vi "Actor Core.vi"(8 "error in":errorcluster, 11 "Nested in":refnum<class "Button_transfer.lvclass">) -> (0 "error out":errorcluster, 3 "Actor out":refnum<class "Actor.lvclass">)   [LabVIEW 2025, in "Button_transfer.lvlib" / "Button_transfer.lvclass"]
doc: "(<B>Filename</B>: Actor Framework.lvlib:Actor.lvclass:Actor Core.vi)\n\nReceives messages to the actor, reacts to them, and initiates any error handling that may shut the actor down.\n\nDescendant classes may override this VI to append parallel tasks for the actor to complete while it handles messages. Overrides use the Call Parent Method node."
uses:
  Button_transfer.lvclass
  C:/Program Files (x86)/National Instruments/LabVIEW 2025/vi.lib/ActorFramework/Actor/Actor.lvclass
  <vilib>/ActorFramework/Actor/Actor.lvclass
  A_Actor/A_Actor.lvclass
  Button_transfer Messages/Update_msg_B Msg/Update_msg_B Msg.lvclass
  C:/Users/halstead_rideriver/Documents/Labview_Practice/Tasks_Actor/A_Actor Messages/A_msg Msg/A_msg Msg.lvclass
  B_Actor/B_Actor.lvclass
  Button_transfer Messages/Update_msg_B2 Msg/Update_msg_B2 Msg.lvclass
  C:/Users/halstead_rideriver/Documents/Labview_Practice/Tasks_Actor/B_Actor Messages/B_msg Msg/B_msg Msg.lvclass
  B_Actor/B_Actor.lvclass/B_Actor.ctl
  A_Actor/A_Actor.lvclass/A_Actor.ctl
  <vilib>/ActorFramework/Actor/Actor.lvclass/Actor.ctl
  <vilib>/ActorFramework/Message Enqueuer/Message Enqueuer.lvclass/Message Enqueuer.ctl
  Button_transfer.lvclass/Button_transfer.ctl
  <vilib>/ActorFramework/Message Enqueuer/Init from Existing Queue.vi
  <vilib>/ActorFramework/Message Enqueuer/Enqueue.vi
  <vilib>/ActorFramework/Stop Msg/Stop Msg.lvclass
  C:/Program Files (x86)/National Instruments/LabVIEW 2025/vi.lib/ActorFramework/Message/Message.lvclass
  <vilib>/ActorFramework/Message Priority Queue/Priority Enqueue.vi
  <vilib>/ActorFramework/Message Enqueuer/Message Enqueuer.lvclass
  C:/Users/halstead_rideriver/Documents/Labview_Practice/Tasks_Actor/Button_transfer/Button_transfer.lvclass
  C:/Users/halstead_rideriver/Documents/Labview_Practice/Tasks_Actor/Button_transfer Messages/Update_msg_B Msg/Update_msg_B Msg.lvclass
  C:/Users/halstead_rideriver/Documents/Labview_Practice/Tasks_Actor/Button_transfer Messages/Update_msg_B2 Msg/Update_msg_B2 Msg.lvclass
  Button_transfer Messages/Generate_no_B Msg/Generate_no_B Msg.lvclass
  C:/Users/halstead_rideriver/Documents/Labview_Practice/Tasks_Actor/B_Actor Messages/Random_B Msg/Random_B Msg.lvclass
  C:/Users/halstead_rideriver/Documents/Labview_Practice/Tasks_Actor/Button_transfer Messages/Generate_no_B Msg/Generate_no_B Msg.lvclass
  C:/Users/halstead_rideriver/Documents/Labview_Practice/Tasks_Actor/A_Actor/A_Actor.lvclass
  C:/Users/halstead_rideriver/Documents/Labview_Practice/Tasks_Actor/B_Actor/B_Actor.lvclass
panel:
  out "Status":string
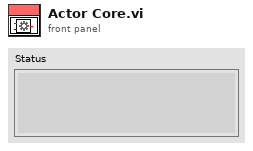
[diagram p1: front panel]
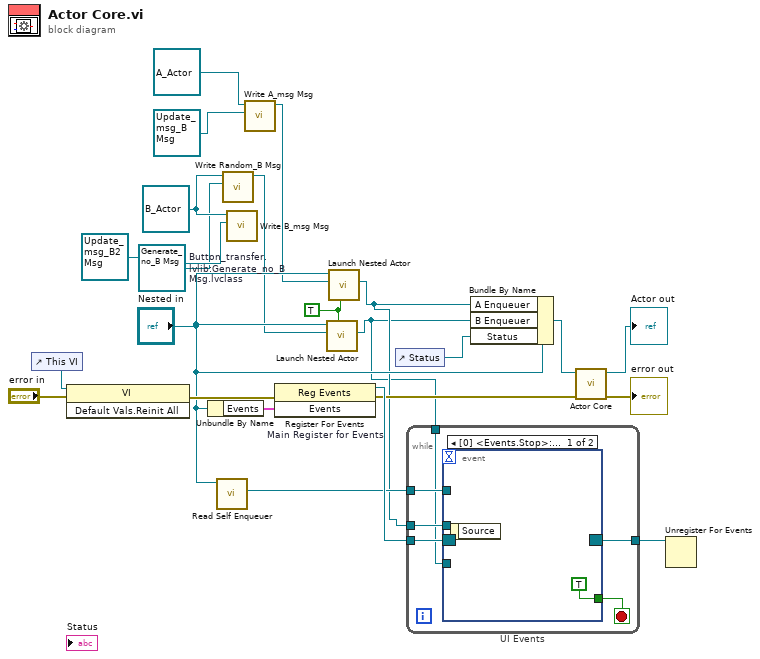
[diagram p0: block diagram]
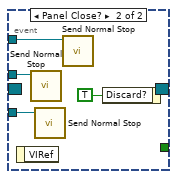
[diagram p2: hidden frame]
diagram:
  w1 = refnum<class "Generate_no_B Msg.lvclass"> refnum  # Button_transfer.lvlib:Generate_no_B Msg.lvclass
  w3 = refnum<class "B_Actor.lvclass"> refnum ("B_Actor.lvlib:B_Actor.lvclass")
  w10 = TRUE ("Open Actor Core front panel? (F)")
  n1 = control-ref of="This VI"() -> (w14:refnum<vi>)
  n2 = invoke class="VI" method="Default Vals.Reinit All"(reference=w14, error in="error in") -> (error out=w12:errorcluster)  [unwired: 1 in, 2 out]
  n3 = Unbundle By Name("Nested in") -> ("Events"=w20:cluster{"Stop":refnum<user-event>})
  n4 = call <vilib>:"Read Self Enqueuer.vi"("Actor"="Nested in") -> ("Self Enqueuer"=w18:refnum<class "Message Enqueuer.lvclass">)  [unwired: 10 in]
  n5 = call "Write Random_B Msg.vi"("B_Actor.lvlib:Random_B Msg.lvclass"=w1, "B_Actor in"=w3) -> ("B_Actor in"=w2:refnum<class "B_Actor.lvclass">)  [unwired: 9 in]
  n6 = call "Write B_msg Msg.vi"("B_Actor.lvlib:B_msg Msg.lvclass"=refnum<class "Update_msg_B2 Msg.lvclass"> refnum ("Button_transfer.lvlib:Update_msg_B2 Msg.lvclass"), "B_Actor in"=w3) -> ()  [unwired: 9 in, 1 out]
  n7 = call "Write A_msg Msg.vi"("A_Actor.lvlib:A_msg Msg.lvclass"=refnum<class "Update_msg_B Msg.lvclass"> refnum ("Button_transfer.lvlib:Update_msg_B Msg.lvclass"), "A_Actor in"=refnum<class "A_Actor.lvclass"> refnum ("A_Actor.lvlib:A_Actor.lvclass")) -> ("A_Actor out"=w5:refnum<class "A_Actor.lvclass">)  [unwired: 9 in]
  n8 = register-events "Main Register for Events"(error in=w12, w20) -> (reference out=w21:refnum<event-registration>, error out=w17:errorcluster)  [unwired: 1 in]
  n9 = call <vilib>:"Launch Nested Actor.vi"("Open Actor Core front panel? (F)"=w10, "Nested Actor"=w2, "Caller Actor in"="Nested in") -> ("Nested Actor's Enqueuer"=w8:refnum<class "Message Enqueuer.lvclass">)  [unwired: 6 in, 2 out]
  n10 = call <vilib>:"Launch Nested Actor.vi"("Open Actor Core front panel? (F)"=w10, "Nested Actor"=w5, "Caller Actor in"="Nested in") -> ("Nested Actor's Enqueuer"=w9:refnum<class "Message Enqueuer.lvclass">)  [unwired: 6 in, 2 out]
  n11 = control-ref of="Status"() -> (w15:refnum<vi>)
  n12 = while {
    tunnel: w21 -> [w29]
    tunnel: [w27] -> w19
    tunnel: w18 -> [w26]
    tunnel: w9 -> [w25]
    tunnel: w8 -> [w24]
    stop <- w28 stop-if-true
    n13 = event "UI Events" shown="[0] <Events.Stop>: User Event" {
      selector: w29 -> [_ _]
      dyn-events: [_ _] -> w27
      timeout: _ -> [_ _]
      tunnel: [TRUE _] -> w28
      tunnel: w26 -> [_ w33]
      tunnel: w25 -> [_ w32]
      tunnel: w24 -> [_ w31]
      event User Event {
        n14 = event-data() -> ()  [unwired: 1 in, 1 out]
      }
      event Panel Close? {
        n15 = event-data() -> ()  [unwired: 1 in, 1 out]
        n16 = call <vilib>:"Send Normal Stop.vi"("Message Enqueuer"=w32) -> ()  [unwired: 10 in, 1 out]
        n17 = call <vilib>:"Send Normal Stop.vi"("Message Enqueuer"=w31) -> ()  [unwired: 10 in, 1 out]
        n18 = call <vilib>:"Send Normal Stop.vi"("Message Enqueuer"=w33) -> ()  [unwired: 10 in, 1 out]
        n19 = event-data("Discard?"=TRUE) -> ()  [unwired: 1 in, 1 out]
      }
    }
  }
  n20 = Bundle By Name(cluster="Nested in", "A Enqueuer"=w9, "B Enqueuer"=w8, "Status"=w15) -> (w16:refnum<class "Button_transfer.lvclass">)
  n21 = call-parent "Actor Core.vi"("error in"=w17, "Actor in"=w16) -> ("error out"=→"error out":errorcluster, "Actor out"=→"Actor out":refnum<class "Actor.lvclass">)  [unwired: 8 in]
  n22 = Unregister For Events(event registration refnum=w19) -> ()  [unwired: 1 in, 1 out]
